vi "Ej 18 DerechaIzquierdaDAQ.vi"() -> ()   [LabVIEW 2021]
uses:
  <vilib>/Instr/_visa.llb/VISA Configure Serial Port (Instr).vi
panel:
  in  "VISA resource name":refnum<visa-resource-name>
  in  "stop":bool
  in  "Duty Cycle (%)":dbl=50.0
  out "Waveform Graph":dynamicdata(graph)
  out "concatenated string":string
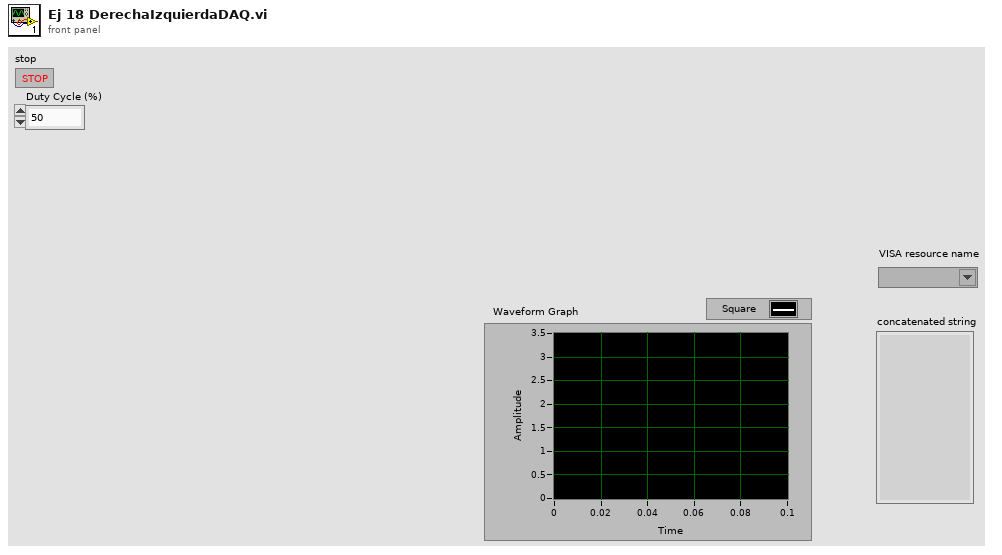
[diagram p1: front panel]
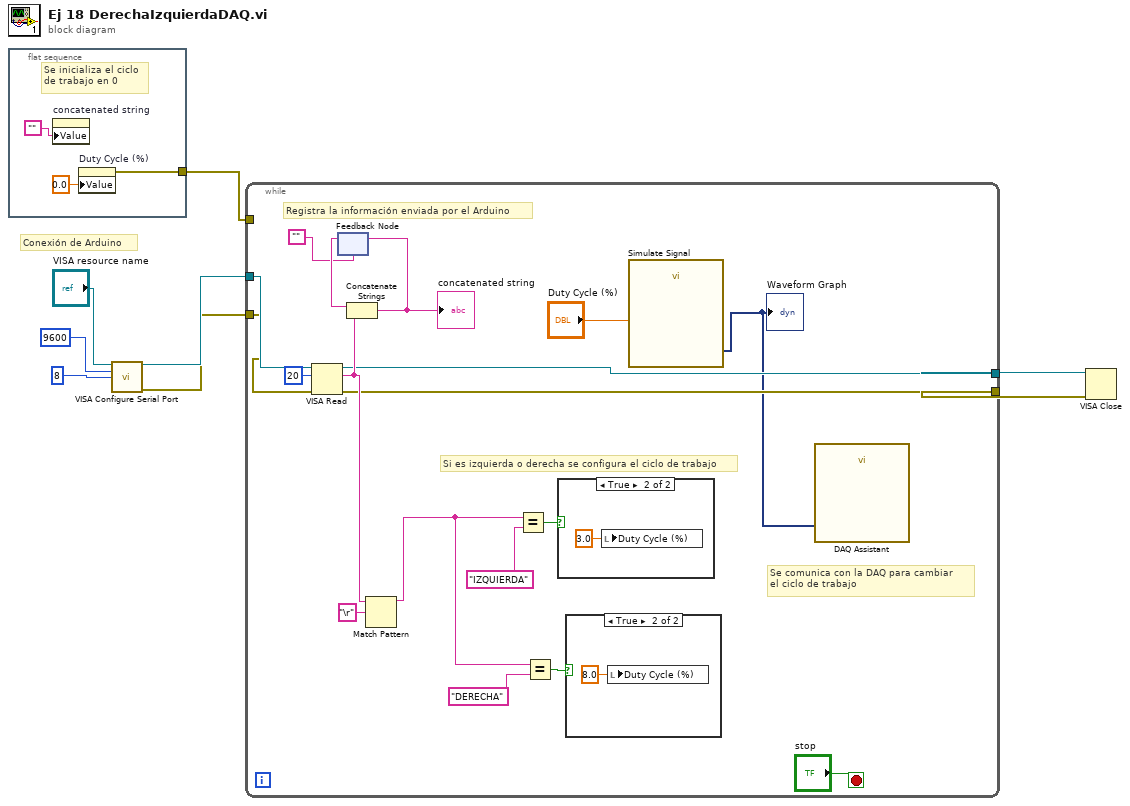
[diagram p0: block diagram]
diagram:
  # "Conexión de Arduino"
  n1 = flat-sequence {
    tunnel: [w9] -> w3
    frame #0 {
      # "Se inicializa el ciclo \nde trabajo en 0"
      n2 = property on="concatenated string" class="Str"("Value"="") -> ()  [unwired: 2 in, 2 out]
      n3 = property on="Duty Cycle (%)" class="DigNum (strict)"("Value"=0.0 ("Duty Cycle (%)")) -> (error out=w9:errorcluster)  [unwired: 2 in, 1 out]
    }
  }
  n4 = call-poly "VISA Configure Serial Port"("VISA resource name"="VISA resource name", "baud rate (9600)"=u32 9600, "data bits (8)"=u16 8) -> ("VISA resource name out"=w8:refnum<visa-resource-name>, "error out"=w7:errorcluster)  [unwired: 11 in]
  n5 = while {
    tunnel: w8 -> [w18]
    tunnel: w7 -> [w17]
    tunnel: [w14] -> w2
    tunnel: w3 -> [_]
    tunnel: [w13] -> w1
    stop <- "stop" stop-if-true
    # "Se comunica con la DAQ para cambiar\nel ciclo de trabajo"
    # "Si es izquierda o derecha se configura el ciclo de trabajo"
    # "Registra la información enviada por el Arduino"
    n6 = VISA Read(VISA resource name=w18, byte count=u32 20, error in (no error)=w17) -> (VISA resource name out=w13:refnum<visa-resource-name>, read buffer=w15:string, error out=w14:errorcluster)  [unwired: 1 out]
    n7 = feedback #1("") -> (w26:string)
    n8 = Concatenate Strings(w26, w15) -> (w27:string)
    "concatenated string" <- w27
    n9 = feedback-in #1(w27) -> ()
    n10 = Match Pattern(string=w15, regular expression="\r") -> (before substring=w22:string)  [unwired: 1 in, 3 out]
    n11 = Equal?(x=w22, y="IZQUIERDA") -> (x = y?=w24:bool)
    n12 = Equal?(x=w22, y="DERECHA") -> (x = y?=w23:bool)
    n13 = case shown="True" w24 {
      frame False {
      }
      frame True {
        n14 = local write "Duty Cycle (%)"(3.0 ("Duty Cycle (%)")) -> ()
      }
    }
    n15 = case shown="True" w23 {
      frame False {
      }
      frame True {
        n16 = local write "Duty Cycle (%)"(8.0 ("Duty Cycle (%)")) -> ()
      }
    }
    n17 = call "Simulate Signal"("Duty Cycle (%)"="Duty Cycle (%)") -> ("Square"=w12:dynamicdata)  [unwired: 13 in, 1 out]
    "Waveform Graph" <- w12
    n18 = call "DAQ Assistant"("data"=w12) -> ()  [unwired: 17 in, 2 out]
  }
  n19 = VISA Close(VISA resource name=w1, error in (no error)=w2) -> ()  [unwired: 1 out]
